vi "Get Path Regex.vi"(8 "error in (no error)":errorcluster, 11 "TestQueryParamController in":refnum<class "TestQueryParamController.lvclass">) -> (0 "error out":errorcluster, 2 "Path Regex":string, 3 "TestQueryParamController out":refnum<class "TestQueryParamController.lvclass">)   [LabVIEW 2020, in "TestQueryParamController.lvclass"]
uses:
  TestQueryParamController.lvclass
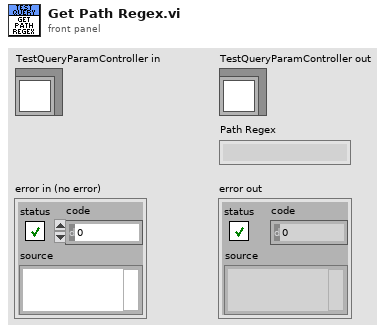
[diagram p1: front panel]
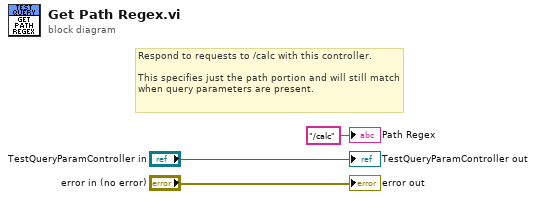
[diagram p0: block diagram]
diagram:
  # "Respond to requests to /calc with this controller.\n\nThis specifies just the path portion and will still match when query parameters are present."
  "error out" <- "error in (no error)"
  "TestQueryParamController out" <- "TestQueryParamController in"
  "Path Regex" <- "/calc" ("Path Regex")
